vi "Return_array.vi"(8 "error in (no error)":errorcluster, 10 "String":string, 11 "JKI_Python_Server in":refnum<class "Server.lvclass">) -> (0 "error out":errorcluster, 3 "JKI_Python_Server out":refnum<class "Server.lvclass">, 7 "Client Connected":bool)   [LabVIEW 2022 SP3]
uses:
  <vilib>/addons/_jki/python_bridge/Server/Server.lvclass
  303f235d-b2b7-4d3d-96b2-58cf21ef0f33.vi
  d3cf6f6b-a4fd-42ef-8031-03215f8826f1.vi
  <vilib>/addons/_jki/python_bridge/Server/Register for Events (Single PyObject).vi
  <vilib>/addons/_jki/python_bridge/Call/Send Return Value.vi
  <vilib>/addons/_jki/python_bridge/Call/Call.lvclass
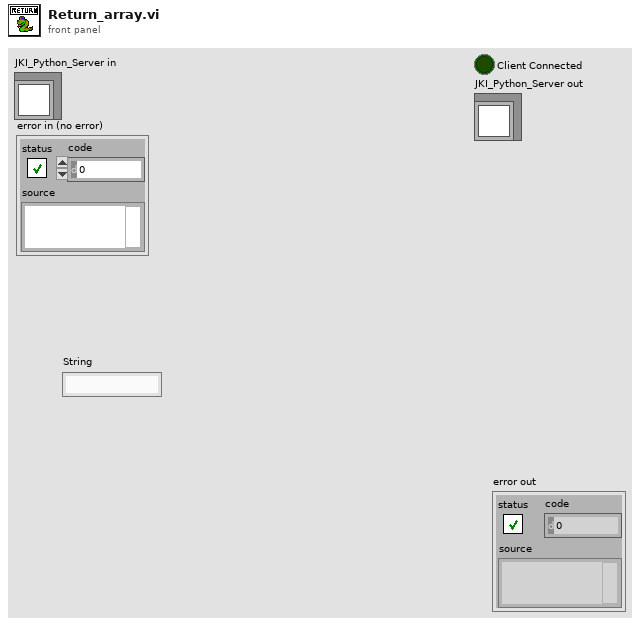
[diagram p1: front panel]
types:
  T1 = cluster{string, "Arguments":string[], "Documentation":string}
  T2 = cluster{string, "Arguments":string[], "Documentation":string}[]
  T3 = typedef "jki_python_bridge.lvlib/Server.lvclass/Python Method Call - Event Registration.ctl" = refnum<event-registration>
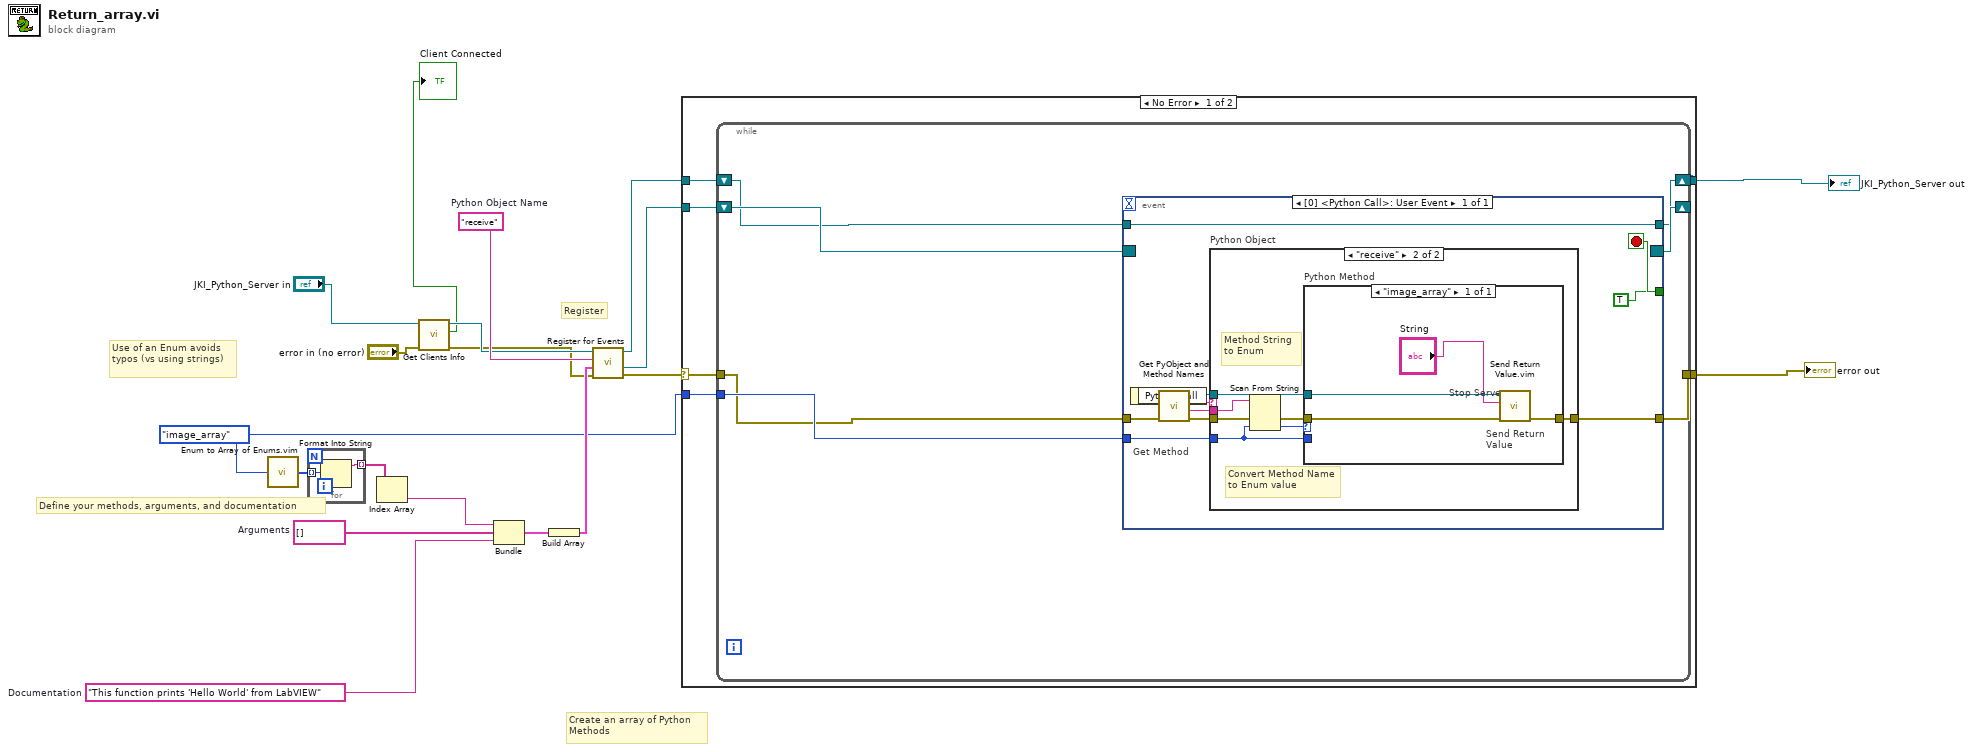
[diagram p0: block diagram]
diagram:
  w12 = string[] []  # Arguments
  w13 = "This function prints 'Hello World' from LabVIEW"  # Documentation
  w11 = enum16{"image_array"}."image_array"
  w19 = "receive"  # Python Object Name
  # "Create an array of Python \nMethods"
  # "Define your methods, arguments, and documentation"
  # "Register"
  # "Use of an Enum avoids typos (vs using strings)"
  n1 = call "Enum to Array of Enums.vim"("enum"=w11) -> ("array of enums"=w10:enum16{"image_array"}[])
  n2 = for {
    tunnel: w10 -> [w21] mode=indexing
    tunnel: [w20] -> w9 mode=indexing
    n3 = Format Into String(w21) -> (resulting string=w20:string)  [unwired: 3 in, 1 out]
  }
  n4 = Index Array(array=w9) -> (element=w16:string)  [unwired: 1 in]
  n5 = call <vilib>:"Get Clients Info.vi"("error in (no error)"="error in (no error)", "JKI_Python_Server in"="JKI_Python_Server in") -> ("error out"=w4:errorcluster, "Client Connected"=→"Client Connected":bool, "JKI_Python_Server out"=w5:refnum<class "Server.lvclass">)  [unwired: 5 in, 2 out]
  n6 = Bundle(w16, "Arguments"=w12, "Documentation"=w13) -> (w15:T1)  [unwired: 1 in]
  n7 = Build Array(w15) -> (w14:T2)
  n8 = call-poly <vilib>:"Register for Events.vi"("error in (no error)"=w4, "Functions"=w14, "PyObject Name"=w19, "JKI_Python_Server in"=w5) -> ("error out"=w8:errorcluster, "Python"=w18:T3, "JKI_Python_Server out"=w17:refnum<class "Server.lvclass">)  [unwired: 5 in]
  n9 = case shown="No Error" w8 {
    selector: w8 -> [w24 w58]
    tunnel: [w27 w59] -> w7
    tunnel: [w26 w58] -> w6
    tunnel: w11 -> [w25 _]
    tunnel: w18 -> [w23 _]
    tunnel: w17 -> [w22 w59]
    frame No Error {
      # "Stop Server"
      n10 = while {
        shift-right: [w31] -> w27
        shift-left: w22 -> [w29]
        shift-right: [w34] -> _
        shift-left: w23 -> [w35]
        tunnel: w25 -> [w33]
        tunnel: w24 -> [w28]
        tunnel: [w32] -> w26
        stop <- w30 stop-if-true
        n11 = event shown="[0] <Python Call>: User Event" {
          selector: w35 -> [_]
          dyn-events: [_] -> w34
          timeout: _ -> [_]
          tunnel: [w39] -> w32
          tunnel: w28 -> [w43]
          tunnel: w29 -> [w45]
          tunnel: [w45] -> w31
          tunnel: w33 -> [w40]
          tunnel: [TRUE] -> w30
          event User Event {
            # "Get Method"
            n12 = event-data() -> ("Python Call"=w44:refnum<class "Call.lvclass">)  [unwired: 1 in]
            n13 = call <vilib>:"Get PyObject and Method Names.vi"("error in (no error)"=w43, "Call in"=w44) -> ("error out"=w42:errorcluster, "Method Name"=w38:string, "PyObject Name"=w37:string, "Call out"=w41:refnum<class "Call.lvclass">)  [unwired: 5 in, 1 out]
            n14 = case "Python Object" shown="\"receive\"" w37 {
              tunnel: w42 -> [w46 w48]
              tunnel: w41 -> [_ w52]
              tunnel: w40 -> [_ w51]
              tunnel: [w46 w50] -> w39
              tunnel: w38 -> [_ w49]
              frame Default {
              }
              frame "receive" {
                # "Convert Method Name to Enum value"
                # "Method String to Enum"
                n15 = Scan From String(input string=w49, error in=w48, default 1=w51) -> (error out=w47:errorcluster, output 1=w53:enum16{"image_array"})  [unwired: 2 in, 2 out]
                n16 = case "Python Method" shown="\"image_array\"" w53 {
                  tunnel: w47 -> [w57]
                  tunnel: [w56] -> w50
                  tunnel: w52 -> [w55]
                  tunnel: w51 -> [_]
                  frame "image_array" {
                    # "Send Return\nValue"
                    n17 = call "Send Return Value.vim"("error in (no error)"=w57, "Return Value"="String", "Response in"=w55) -> ("error out"=w56:errorcluster)  [unwired: 8 in]
                  }
                }
              }
            }
          }
        }
      }
    }
    frame Error {
    }
  }
  "JKI_Python_Server out" <- w7
  "error out" <- w6
